vi "Validate Config.vi"(10 "VolatusConfig":refnum<class "VolatusConfig.lvclass">) -> (0 "error out":errorcluster)   [LabVIEW 2020, in "VolatusConfig.lvlib"]
uses:
  VolatusConfig.lvlib
  VolatusConfig/VolatusConfig.lvclass
  VolatusErrorUtilities/MultiErrors/MultiErrors.lvclass
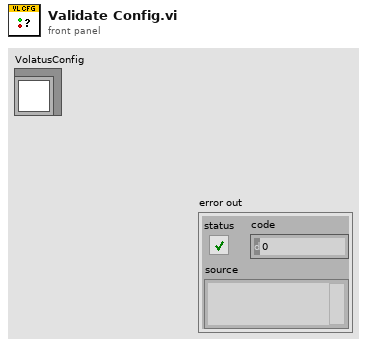
[diagram p1: front panel]
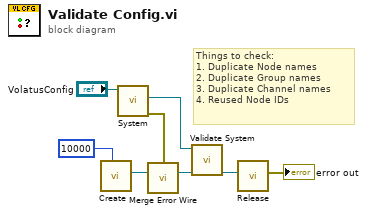
[diagram p0: block diagram]
diagram:
  # "Things to check:\n1. Duplicate Node names\n2. Duplicate Group names\n3. Duplicate Channel names\n4. Reused Node IDs"
  n1 = call "Create.vi"("Max Errors (200)"=10000) -> ("MultiErrors out"=w7:refnum<class "MultiErrors.lvclass">)  [unwired: 10 in]
  n2 = call "System.vi"("VolatusConfig in"="VolatusConfig") -> ("error out"=w1:errorcluster, "System"=w2:refnum<class "System Config.lvclass">)  [unwired: 8 in, 1 out]
  n3 = call "Merge Error Wire.vi"("error in (no error)"=w1, "MultiErrors in"=w7) -> ("MultiErrors out"=w6:refnum<class "MultiErrors.lvclass">)  [unwired: 13 in]
  n4 = call "Validate System.vi"("errors in"=w6, "System Config"=w2) -> ("errors out"=w5:refnum<class "MultiErrors.lvclass">)  [unwired: 9 in]
  n5 = call "Release.vi"("MultiErrors in"=w5) -> ("error out"=→"error out":errorcluster)  [unwired: 10 in]
